vi "UIRef.vi"(8 "error in":errorcluster, 11 "Standard Engine in":refnum<class "Standard Engine Editor Node.lvclass">=refnum) -> (0 "error out":errorcluster, 2 "VI refnum":refnum<vi>, 3 "Standard Engine out":refnum<class "Standard Engine Editor Node.lvclass">)   [LabVIEW 2013, in "Standard Engine Editor Node.lvclass"]
doc: "Stores the static reference to the UI of the node."
uses:
  Standard Engine Editor Node.lvclass
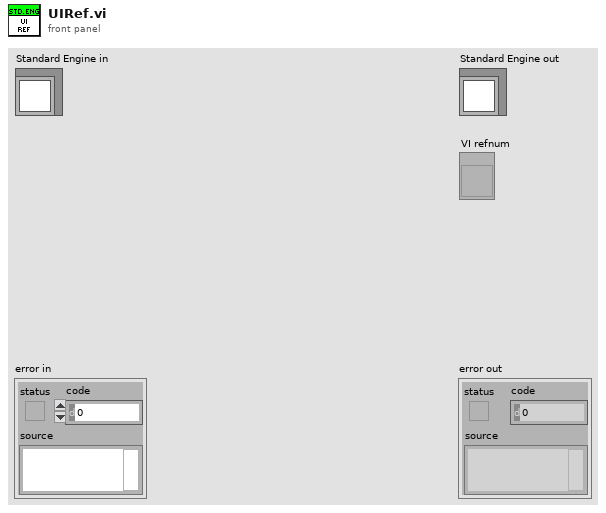
[diagram p1: front panel]
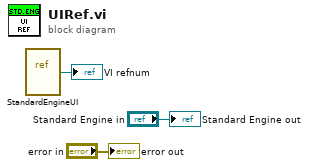
[diagram p0: block diagram]
diagram:
  n1 = vi-ref "StandardEngineUI.vi"() -> (→"VI refnum":refnum<vi>)
  "error out" <- "error in"
  "Standard Engine out" <- "Standard Engine in"
